vi "RX-ADAR-TEMP.vi"(0 "COMPORT":refnum<visa-resource-name>="COM4", 7 "RevC(t)":bool=TRUE, 11 "error in (no error)":errorcluster, 12 "RxPort":i32, 13 "Open/Close Serial":bool) -> (2 "All Success":bool=TRUE, 4 "comport":refnum<visa-resource-name>="COM4", 8 "temp(c)":dbl=23.950000000000003, 15 "error out":errorcluster)   [LabVIEW 2018]
panel:
  out "cmd":string
  out "after substring":string="63\r\n>\r\n"
  out "output 2":string="\rwr rxm 0x30 0x70\r\n>\rrd rxm 0x31\r\n0x031: 0x63\r\n>"
  out "string":string="wr rxm 0x30 0x70\r\n>\nrd rxm 0x31\r\n0x031: 0x63\r\n>\r\n"
  out "Success":bool[](array[boolean])=[TRUE, TRUE]
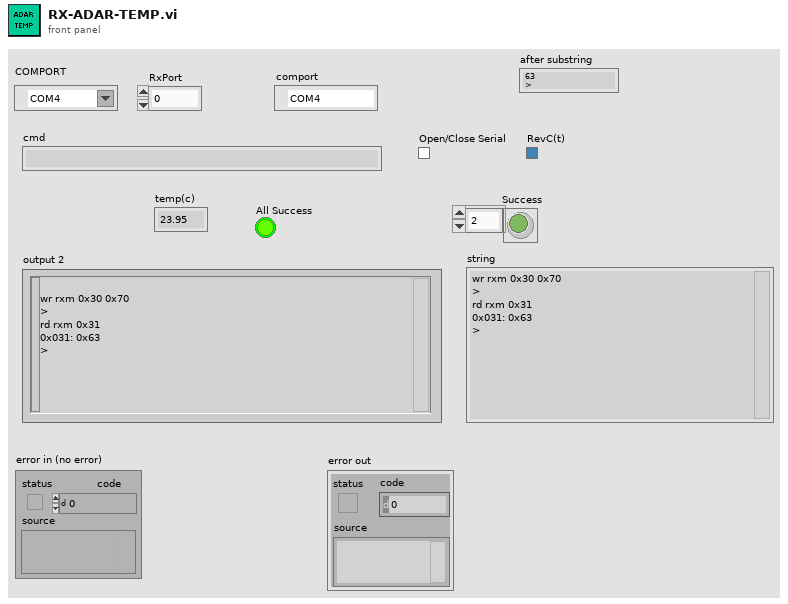
[diagram p1: front panel]
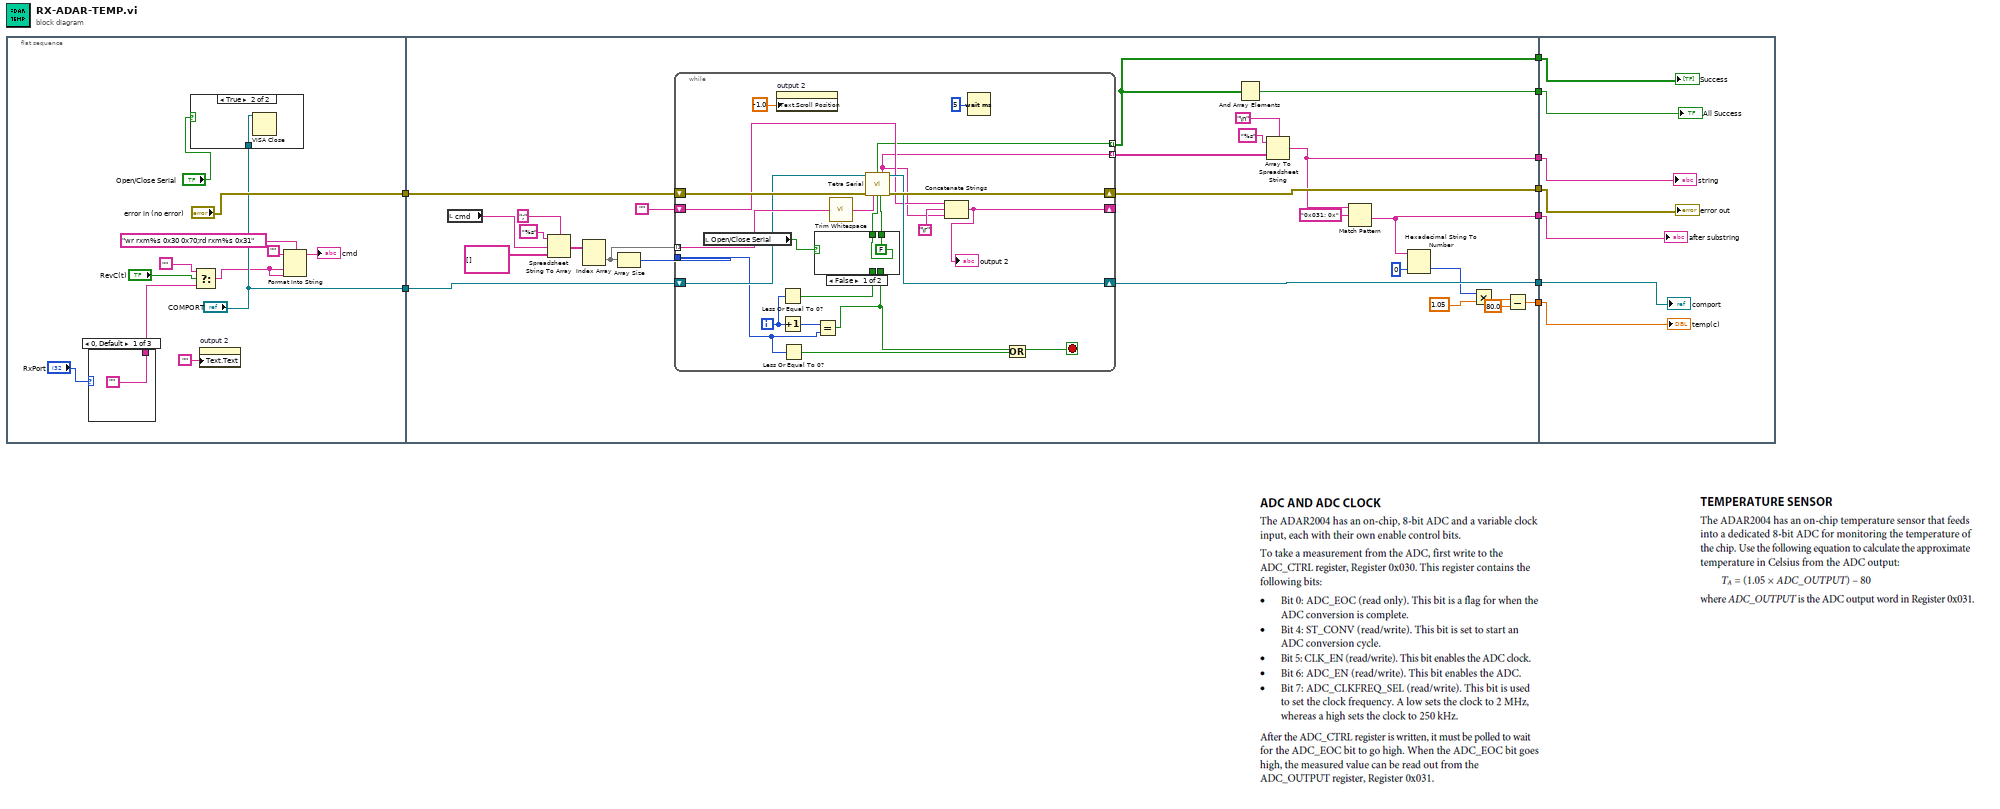
[diagram p0: block diagram]
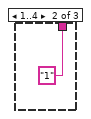
[diagram p2: hidden frame]
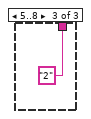
[diagram p3: hidden frame]
diagram:
  n1 = flat-sequence {
    tunnel: ["error in (no error)"] -> w2
    tunnel: ["COMPORT"] -> w1
    tunnel: [w47] -> w9
    tunnel: [w44] -> w8
    tunnel: [w39] -> w7
    tunnel: [w38] -> w6
    tunnel: [w35] -> w5
    tunnel: [w33] -> w4
    tunnel: [w27] -> w3
    tunnel: w2 -> [w46]
    tunnel: w1 -> [w45]
    tunnel: w9 -> [w78]
    tunnel: w8 -> [w79]
    tunnel: w7 -> [w80]
    tunnel: w6 -> [w82]
    tunnel: w5 -> [w81]
    tunnel: w4 -> [w83]
    tunnel: w3 -> [w84]
    frame #0 {
      n2 = case shown="0, Default" "RxPort" {
        tunnel: ["" "1" ("f") "2" ("f")] -> w13
        frame 0, Default {
        }
        frame 1..4 {
        }
        frame 5..8 {
        }
      }
      n3 = case shown="True" "Open/Close Serial" {
        tunnel: "COMPORT" -> [_ w25]
        frame False {
        }
        frame True {
          n4 = VISA Close(VISA resource name=w25) -> ()  [unwired: 1 in, 1 out]
        }
      }
      n5 = Select(t="", s="RevC(t)", f=w13) -> (s? t:f=w11:string)
      n6 = property on="output 2" class="Str"("Text.Text"="") -> ()  [unwired: 2 in, 2 out]
      n7 = Format Into String(format string="wr rxm%s 0x30 0x70;rd rxm%s 0x31" ("Command ( ; seperation)"), initial string="", w11, w11) -> (resulting string=→"cmd":string)  [unwired: 1 in, 1 out]
    }
    frame #1 {
      n8 = local read "cmd"() -> (w26:string)
      n9 = Spreadsheet String To Array(delimiter (Tab)=";", format string="%s", spreadsheet string=w26, array type (2D Dbl)=string[][] []) -> (array=w48:string[][])
      n10 = Index Array(array=w48) -> (element=w43:string[])  [unwired: 2 in]
      n11 = Array Size(array=w43) -> (size(s)=w36:i32)
      n12 = while {
        shift-right: [w74] -> w47
        shift-left: w46 -> [w73]
        shift-right: [w72] -> w44
        shift-left: w45 -> [w61]
        tunnel: [w67] -> w37 mode=indexing
        tunnel: w43 -> [w71] mode=indexing
        tunnel: w36 -> [w59]
        shift-right: [w64] -> _
        shift-left: "" -> [w68]
        tunnel: [w65] -> w39 mode=indexing
        i -> [w62]
        stop <- w60 stop-if-true
        n13 = local read "Open/Close Serial"() -> (w52:bool)
        n14 = property on="output 2" class="Str"("Text.Scroll Position"=-1.0) -> ()  [unwired: 2 in, 2 out]
        n15 = Less Or Equal To 0?(x=w62) -> (x <= 0?=w55:bool)
        n16 = Increment(x=w62) -> (x+1=w63:i32)
        n17 = Less Or Equal To 0?(x=w59) -> (x <= 0?=w58:bool)
        n18 = Equal?(x=w63, y=w59) -> (x = y?=w54:bool)
        n19 = case shown="False" w52 {
          tunnel: [w75 w77] -> w56
          tunnel: w55 -> [_ w77]
          tunnel: w54 -> [_ w76]
          tunnel: [w75 w76] -> w53
          frame False {
            w75 = FALSE
          }
          frame True {
          }
        }
        n20 = call <vilib>:"Trim Whitespace.vi"("string"=w71) -> ("trimmed string"=w66:string)  [unwired: 1 in]
        n21 = call "Tetra Serial.vi"("COMPORT"=w61, "error in (no error)"=w73, "Command"=w66, "Open Ser(t)"=w56, "Close Ser(t)"=w53) -> ("Success"=w65:bool, "output"=w67:string, "comport"=w72:refnum<visa-resource-name>, "error out"=w74:errorcluster)  [unwired: 6 in, 1 out]
        n22 = Concatenate Strings(w68, "\r", w67) -> (w64:string)
        "output 2" <- w64
        n23 = Wait (ms)(milliseconds to wait=u32 5) -> ()  [unwired: 1 out]
        n24 = Or(x=w54, y=w58) -> (x .or. y?=w60:bool)
      }
      n25 = And Array Elements(Boolean array=w39) -> (logical AND=w38:bool)
      n26 = Array To Spreadsheet String(delimiter (Tab)="\n", array=w37, 3:"%s" ("format string")) -> (spreadsheet string=w35:string)
      n27 = Match Pattern(string=w35, regular expression="0x031: 0x") -> (after substring=w33:string)  [unwired: 1 in, 3 out]
      n28 = Hexadecimal String To Number(string=w33, default (0uL)=0 ("default (0 U32)")) -> (number=w31:i32)  [unwired: 1 in, 1 out]
      n29 = Multiply(x=w31, y=1.05) -> (x*y=w29:dbl)
      n30 = Subtract(x=w29, y=80.0) -> (x-y=w27:dbl)
    }
    frame #2 {
      "error out" <- w78
      "comport" <- w79
      "Success" <- w80
      "string" <- w81
      "All Success" <- w82
      "after substring" <- w83
      "temp(c)" <- w84
    }
  }
